vi "Global.vi"() -> ()   [LabVIEW 2021]
panel:
  in  "有源音箱":bool
  in  "扫频模式":bool
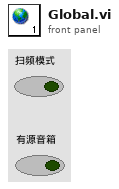
[diagram p1: front panel]
diagram:
